vi "Find all Classes in LV XML.vi"(8 "error in (no error)":errorcluster, 11 "Project Path":path) -> (0 "error out":errorcluster, 3 "Class Paths":path[](array[path]))   [LabVIEW 2020, in "Test Finder.lvclass"]
uses:
  Test Finder.lvclass
  Test Finder.lvclass/Test Finder.ctl
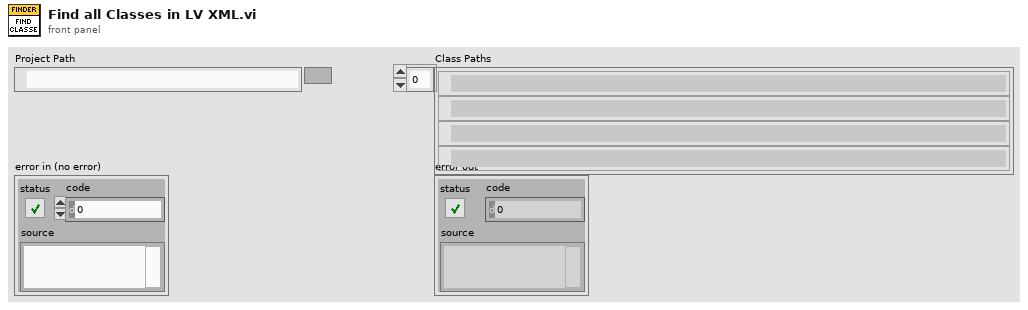
[diagram p1: front panel]
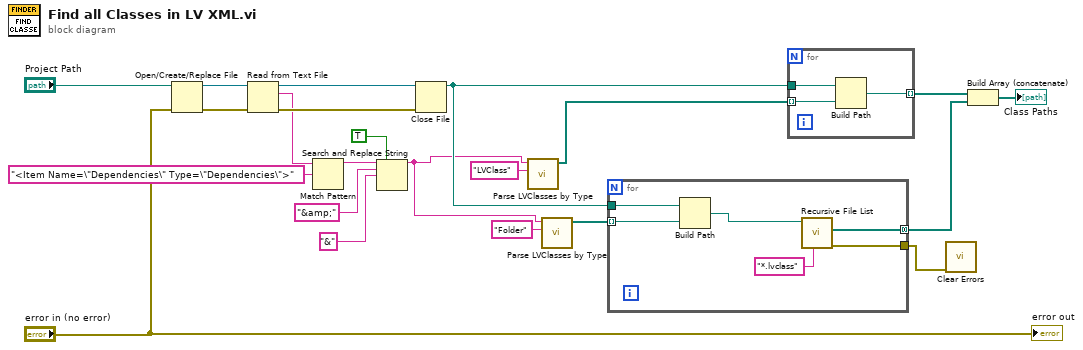
[diagram p0: block diagram]
diagram:
  n1 = Open/Create/Replace File(file path (use dialog)="Project Path", error in="error in (no error)") -> (refnum out=w22:refnum<file>, error out=w21:errorcluster)  [unwired: 4 in, 1 out]
  n2 = Read from Text File(file (use dialog)=w22, error in=w21) -> (refnum out=w20:refnum<file>, text=w6:string, error out=w19:errorcluster)  [unwired: 2 in, 1 out]
  n3 = Match Pattern(string=w6, regular expression="<Item Name=\"Dependencies\" Type=\"Dependencies\">") -> (before substring=w5:string)  [unwired: 1 in, 3 out]
  n4 = Search and Replace String(replace all?=TRUE ("replace all? (F)"), input string=w5, search string="&amp;", replace string="&" ("search string")) -> (result string=w4:string)  [unwired: 4 in, 3 out]
  n5 = Close File(refnum=w20, error in=w19) -> (path=w8:path)  [unwired: 1 out]
  n6 = call "Parse LVClasses by Type.vi"("Type"="LVClass", "Input"=w4) -> ("Relative Paths"=w18:path[])  [unwired: 9 in]
  n7 = call "Parse LVClasses by Type.vi"("Type"="Folder", "Input"=w4) -> ("Relative Paths"=w12:path[])  [unwired: 9 in]
  n8 = for {
    tunnel: w12 -> [w23] mode=indexing
    tunnel: [w27] -> w11 mode=concatenating
    tunnel: [w26] -> w10
    tunnel: w8 -> [w25]
    n9 = Build Path(base path=w25, name or relative path=w23) -> (appended path=w24:path)
    n10 = call <vilib>:"Recursive File List.vi"("pattern"="*.lvclass", "Folder Path"=w24) -> ("error out"=w26:errorcluster, "All Files in Dir"=w27:path[])  [unwired: 5 in, 3 out]
  }
  n11 = for {
    tunnel: w8 -> [w31]
    tunnel: w18 -> [w30] mode=indexing
    tunnel: [w29] -> w17 mode=indexing
    n12 = Build Path(base path=w31, name or relative path=w30) -> (appended path=w29:path)
  }
  n13 = call <vilib>:"Clear Errors.vi"("error in (no error)"=w10) -> ()  [unwired: 5 in, 2 out]
  n14 = Build Array (concatenate)(w17, w11) -> (→"Class Paths":path[])
  "error out" <- "error in (no error)"
